vi "Read DAQmx Pulse Settings.vi"(11 "DAQmx_pulse_out in":refnum<class "DAQmx_DO.lvclass">) -> (2 "DAQmx Pulse Settings":T1={"Enable DAQmx Pulses"=FALSE, "DAQmx Physical Channels"="Dev2/port0_32", "Clock Rate"=10000000.0, "units/sec (ms=1000)"=1000.0, "Start Trigger"={"Wait for start trigger?"=FALSE, "source"="/Dev1/PFI0", "edge"=10280}, "waveform"={"name"="", "transitions"=[], "states"=[]}} {"Start Trigger"."edge" items=["Rising"=10280, "Falling"=10171]; "Clock Rate" min=0.0 max=200000000.0 format="%.2p"})   [LabVIEW 2013, in "DAQmx_DO.lvclass"]
uses:
  DAQmx_DO.lvclass
  settings.ctl
  HSDIO/waveform.ctl
  DAQmx_DO.lvclass/DAQmx_DO.ctl
  HSDIO/HSDIO.lvclass
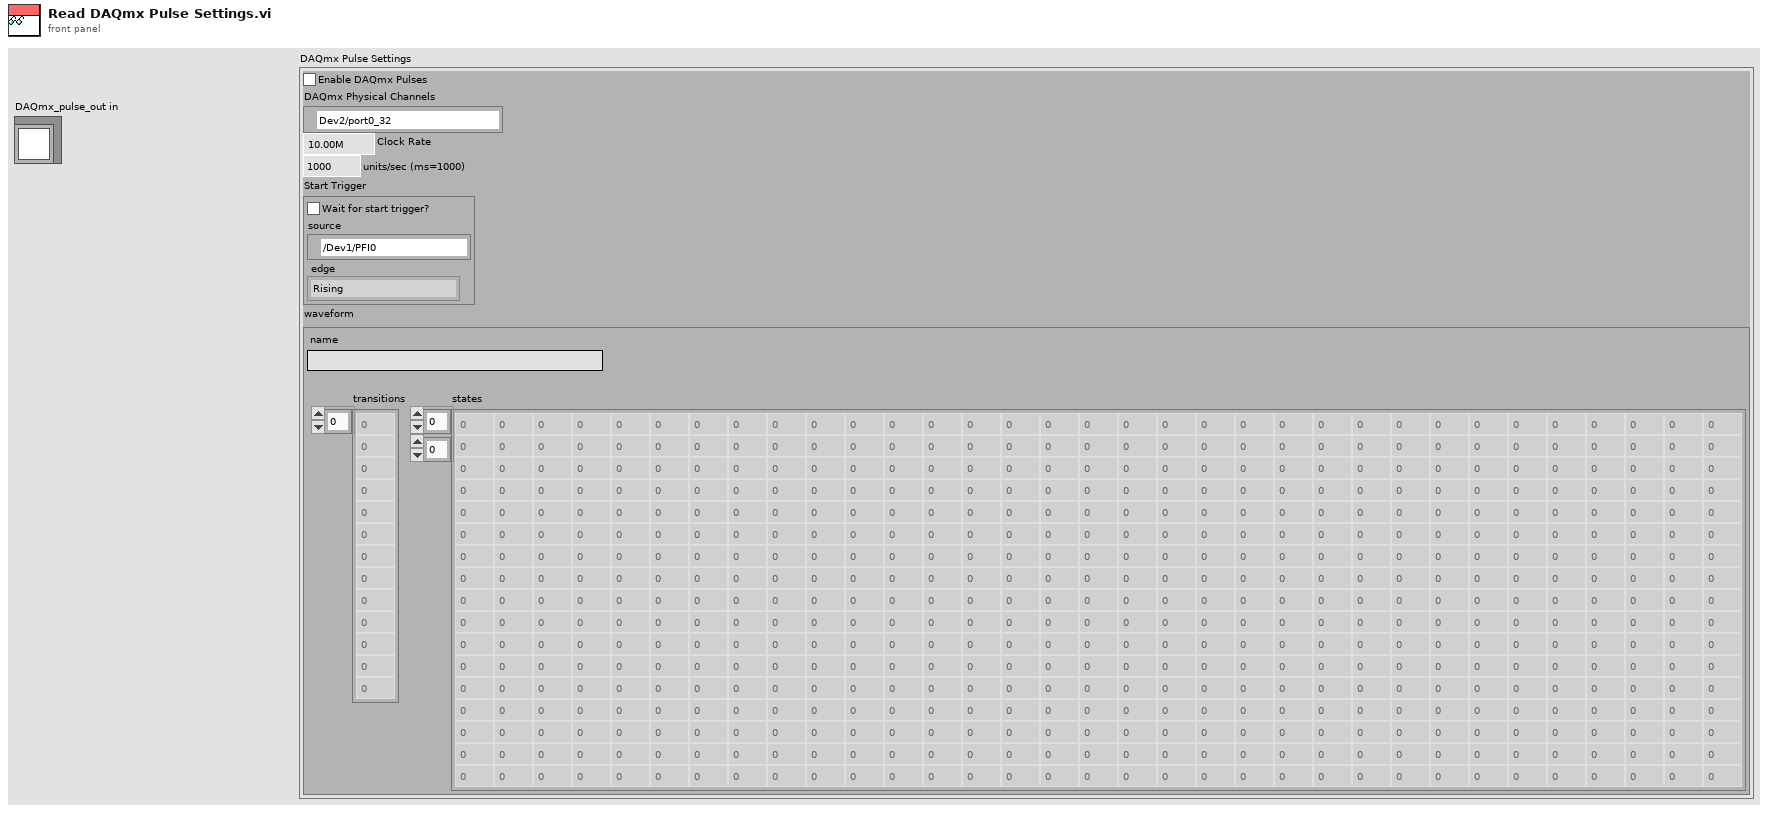
[diagram p1: front panel]
types:
  T1 = typedef "DAQmx_DO.lvclass/settings.ctl" = cluster{"Enable DAQmx Pulses":bool, "DAQmx Physical Channels":tag, "Clock Rate":dbl, "units/sec (ms=1000)":dbl, "Start Trigger":cluster{"Wait for start trigger?":bool, "source":tag, "edge":i32}, "waveform":T2}
  T2 = typedef "HSDIO.lvclass/waveform.ctl" = cluster{"name":string, "transitions":u32[], "states":u8[][]}
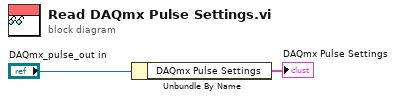
[diagram p0: block diagram]
diagram:
  n1 = Unbundle By Name("DAQmx_pulse_out in") -> ("DAQmx Pulse Settings"=→"DAQmx Pulse Settings":T1)
